vi "BridgeAutoSequence.vi"(8 "error in (no error)":errorcluster, 11 "Auto Start":u32) -> ()   [LabVIEW 2011]
uses:
  <vilib>/Rock Robotics/WPI/Solenoid/WPI_SolenoidValue.ctl
  <vilib>/Rock Robotics/WPI/Solenoid/WPI_SolenoidSetEnum.vi
  <vilib>/Rock Robotics/WPI/Solenoid/Deprecated/WPI_SolenoidSetBool.vi
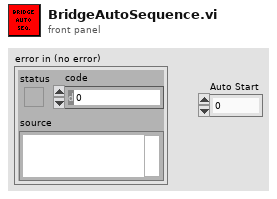
[diagram p1: front panel]
types:
  T1 = typedef "WPI_SolenoidValue.ctl" = enum16{"Off", "On", "Forward", "Reverse"}
  T2 = typedef "WPI_RobotDriveDevRef.ctl" = cluster{"DevStatus":errorcluster, "Motors[]":T3[], "Square Inputs":bool, "Max Output":dbl, "Isochronous":bool}
  T3 = typedef "WPI_MotorControlDeviceRef.ctl" = cluster{"DeviceStatus":errorcluster, "Type":enum16{"PWM", "CAN"}, "PWM":cluster{"Digital Module":T4, "PWM Channel":T5, "DeadBand":T6}, "CAN":cluster{"Device Number":u8, "Control Mode":T7, "Semaphore":T8, "Max Vout":dbl}, "Invert":bool, "TransformRef":T9, "InvTransformRef":T9}
  T4 = typedef "FPGA_TypedefDigitalModule.ctl" = enum16{"Digital Module 1", "Digital Module 2"}
  T5 = typedef "FPGA_DIOPWMChannel.ctl" = enum8{"PWM 1", "PWM 2", "PWM 3", "PWM 4", "PWM 5", "PWM 6", "PWM 7", "PWM 8", "PWM 9", "PWM 10", "Invalid"}
  T6 = typedef "WPI_PWMDeadband.ctl" = cluster{"Name":string, "maxPositivePwm":i32, "minPositivePwm":i32, "centerPwm":i32, "maxNegativePwm":i32, "minNegativePwm":i32, "angularRange":u16}
  T7 = typedef "WPI_CANJaguar_ControlMode.ctl" = enum8{"Percent VBus", "Current", "Speed", "Position", "Voltage"}
  T8 = typedef "Semaphore RefNum" = refnum<k1>
  T9 = typedef "WPI_PWMTransform_ConPane.ctl" = refnum<vi>
  T10 = typedef "WPI_SolenoidDevRef.ctl" = cluster{"DevStatus":errorcluster, "Solenoid Module":T11, "Forward Solenoid Channel":T12, "Reverse Solenoid Channel":T12}
  T11 = typedef "FPGA_TypedefSolenoidModule.ctl" = enum16{"Solenoid Module 1", "Solenoid Module 2"}
  T12 = typedef "WPI_SolenoidChannel.ctl" = enum8{"Solenoid 1", "Solenoid 2", "Solenoid 3", "Solenoid 4", "Solenoid 5", "Solenoid 6", "Solenoid 7", "Solenoid 8", "Invalid"}
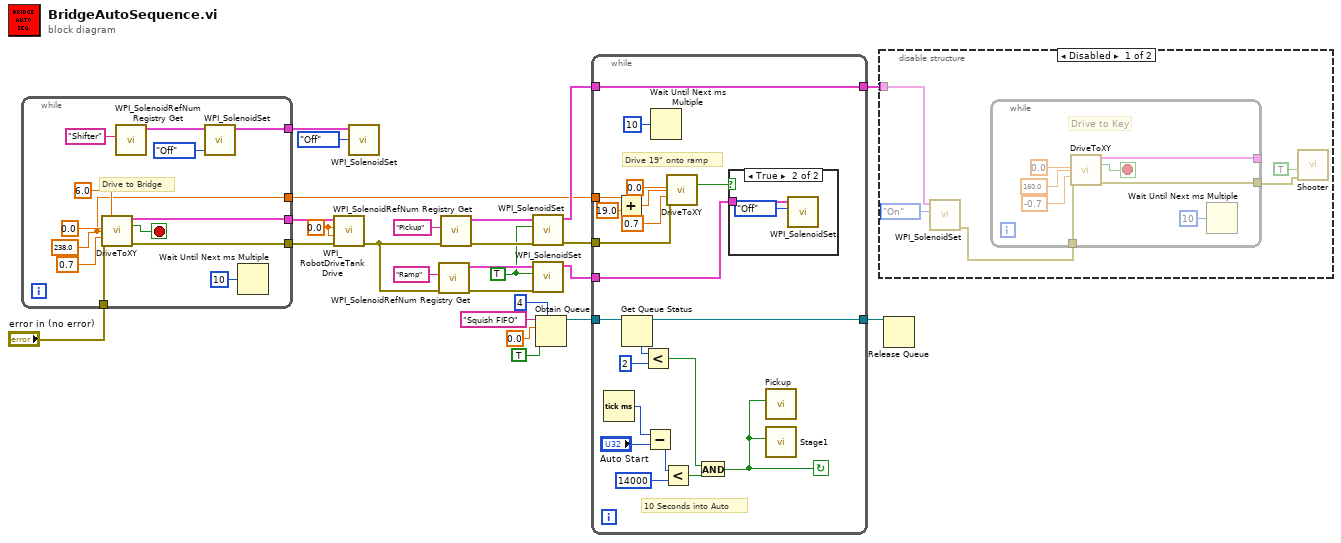
[diagram p0: block diagram]
diagram:
  w2 = TRUE ("x .and. y?")
  w25 = 0.0 ("Left axis value")
  n1 = while {
    tunnel: [w36] -> w24
    tunnel: "error in (no error)" -> [w35]
    tunnel: [w32] -> w23
    tunnel: [w28] -> w9
    tunnel: [w26] -> w1
    stop <- w34 stop-if-true
    w26 = 238.0 ("Y Target")
    # "Drive to Bridge"
    n2 = call "DriveToXY.vi"("Drive Margin"=6.0, "X Target"=0.0, "Y Target"=w26, "Speed"=0.7, "error in"=w35) -> ("RobotDriveDevRef Out"=w32:T2, "At Target"=w34:bool, "error out"=w36:errorcluster)  [unwired: 8 in]
    n3 = call <vilib>:"WPI_SolenoidRefNum Registry Get.vi"("refnum name"="Shifter") -> ("SolenoidDevRef"=w30:T10)  [unwired: 1 in, 9 out]
    n4 = call-poly <vilib>:"WPI_SolenoidSet.vi"("Value"=WPI_SolenoidValue."Off", "SolenoidDevRef"=w30) -> ("SolenoidDevRef"=w28:T10)  [unwired: 1 in, 8 out]
    n5 = Wait Until Next ms Multiple(millisecond multiple=u32 10) -> ()  [unwired: 1 out]
  }
  n6 = call <vilib>:"WPI_RobotDriveTankDrive.vi"("error in (no error)"=w24, "Right axis value"=w25, "Left axis value"=w25, "RobotDriveDevRef"=w23) -> ("error out"=w6:errorcluster)  [unwired: 6 in, 1 out]
  n7 = call-poly <vilib>:"WPI_SolenoidSet.vi"("Value"=WPI_SolenoidValue."Off", "SolenoidDevRef"=w9) -> ()  [unwired: 1 in, 9 out]
  n8 = call <vilib>:"WPI_SolenoidRefNum Registry Get.vi"("error in (no error)"=w6, "refnum name"="Ramp") -> ("error out"=w12:errorcluster, "SolenoidDevRef"=w13:T10)  [unwired: 8 in]
  n9 = call <vilib>:"WPI_SolenoidRefNum Registry Get.vi"("error in (no error)"=w6, "refnum name"="Pickup") -> ("error out"=w14:errorcluster, "SolenoidDevRef"=w15:T10)  [unwired: 8 in]
  n10 = call-poly <vilib>:"WPI_SolenoidSet.vi"("error in (no error)"=w14, "Value"=w2, "SolenoidDevRef"=w15) -> ("error out"=w11:errorcluster, "SolenoidDevRef"=w4:T10)  [unwired: 7 in]
  n11 = call-poly <vilib>:"WPI_SolenoidSet.vi"("error in (no error)"=w12, "Value"=w2, "SolenoidDevRef"=w13) -> ("SolenoidDevRef"=w5:T10)  [unwired: 7 in, 1 out]
  n12 = Obtain Queue(max queue size (-1, unlimited)=4, name (unnamed)="Squish FIFO", element data type=sgl 0.0 ("Voltage"), create if not found? (T)=TRUE) -> (queue out=w18:refnum<queue>)  [unwired: 1 in, 2 out]
  n13 = while {
    tunnel: w18 -> [w59]
    tunnel: w11 -> [w58]
    tunnel: [w57] -> w8
    tunnel: w5 -> [w53]
    tunnel: w4 -> [w52]
    tunnel: [w52] -> w3
    tunnel: w1 -> [w44]
    stop <- w45 continue-if-true
    # "Drive 19\" onto ramp"
    # "10 Seconds into Auto"
    n14 = Tick Count (ms)() -> (millisecond timer value=w48:u32)
    n15 = Add(x=w44, y=19.0) -> (x+y=w40:dbl)
    n16 = Get Queue Status(queue=w59) -> (queue out=w57:refnum<queue>, # elements in queue=w55:i32)  [unwired: 2 in, 6 out]
    n17 = Less?(x=w55, y=2) -> (x < y?=w49:bool)
    n18 = Subtract(x=w48, y="Auto Start") -> (x-y=w47:u32)
    n19 = Wait Until Next ms Multiple(millisecond multiple=u32 10) -> ()  [unwired: 1 out]
    n20 = Less?(x=w47, y=14000) -> (x < y?=w50:bool)
    n21 = call "DriveToXY.vi"("X Target"=0.0, "Y Target"=w40, "Speed"=0.7, "error in"=w58) -> ("At Target"=w41:bool)  [unwired: 9 in, 2 out]
    n22 = And(x=w49, y=w50) -> (x .and. y?=w45:bool)
    n23 = case shown="True" w41 {
      tunnel: w53 -> [_ w60]
      frame False {
      }
      frame True {
        n24 = call-poly <vilib>:"WPI_SolenoidSet.vi"("Value"=WPI_SolenoidValue."Off", "SolenoidDevRef"=w60) -> ()  [unwired: 8 in, 2 out]
      }
    }
    n25 = call "Pickup.vi"("On?"=w45) -> ()  [unwired: 11 in]
    n26 = call "Stage1.vi"("On?"=w45) -> ()  [unwired: 11 in]
  }
  n27 = disable-structure shown="Disabled" {
    disable-tunnel: w3 -> [w64 _]
    frame Disabled {
      n28 = call-poly <vilib>:"WPI_SolenoidSet.vi"("Value"=WPI_SolenoidValue."On", "SolenoidDevRef"=w64) -> ("error out"=w63:errorcluster)  [unwired: 8 in, 1 out]
      n29 = while {
        tunnel: [w71] -> w62
        tunnel: w63 -> [w70]
        tunnel: [w67] -> _
        stop <- w69 stop-if-true
        # "Drive to Key"
        n30 = call "DriveToXY.vi"("X Target"=0.0, "Y Target"=160.0, "Speed"=-0.7, "error in"=w70) -> ("RobotDriveDevRef Out"=w67:T2, "At Target"=w69:bool, "error out"=w71:errorcluster)  [unwired: 9 in]
        n31 = Wait Until Next ms Multiple(millisecond multiple=u32 10) -> ()  [unwired: 1 out]
      }
      n32 = call "Shooter.vi"("error in (no error)"=w62, "Use Camera"=TRUE) -> ()  [unwired: 8 in, 2 out]
    }
    frame Enabled {
    }
  }
  n33 = Release Queue(queue=w8) -> ()  [unwired: 2 in, 3 out]
